vi "parse CSV files.vi"(6 "threshold cases":u32, 7 "SA data":T1, 8 "US data":T1, 9 "deaths CSV":string[][](array[string]), 10 "country index":u16, 11 "cases CSV":string[][](array[string])) -> (0 "new deaths per day":i32[](array[numeric]), 1 "days":i32[](array[numeric]), 2 "new cases per day":i32[](array[numeric]), 3 "first case date":timestamp, 4 "cumulative cases":i32[](array[numeric]), 5 "cumulative deaths":i32[](array[numeric]))   [LabVIEW 2019]
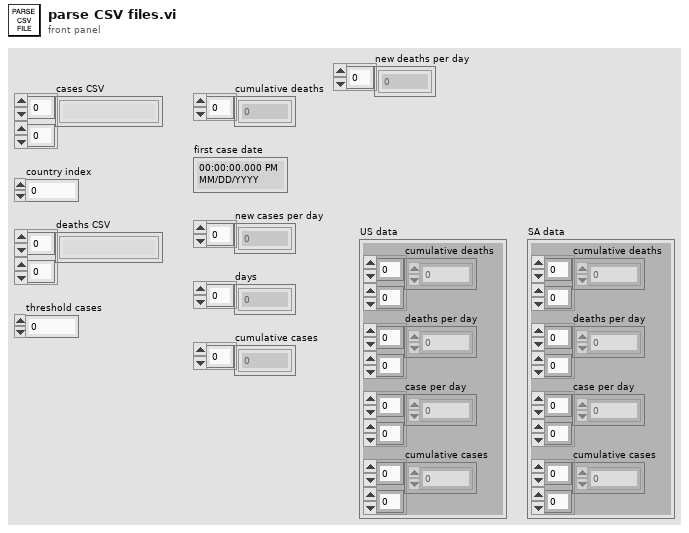
[diagram p1: front panel]
types:
  T1 = cluster{"cumulative deaths":i32[][], "deaths per day":i32[][], "case per day":i32[][], "cumulative cases":i32[][]}
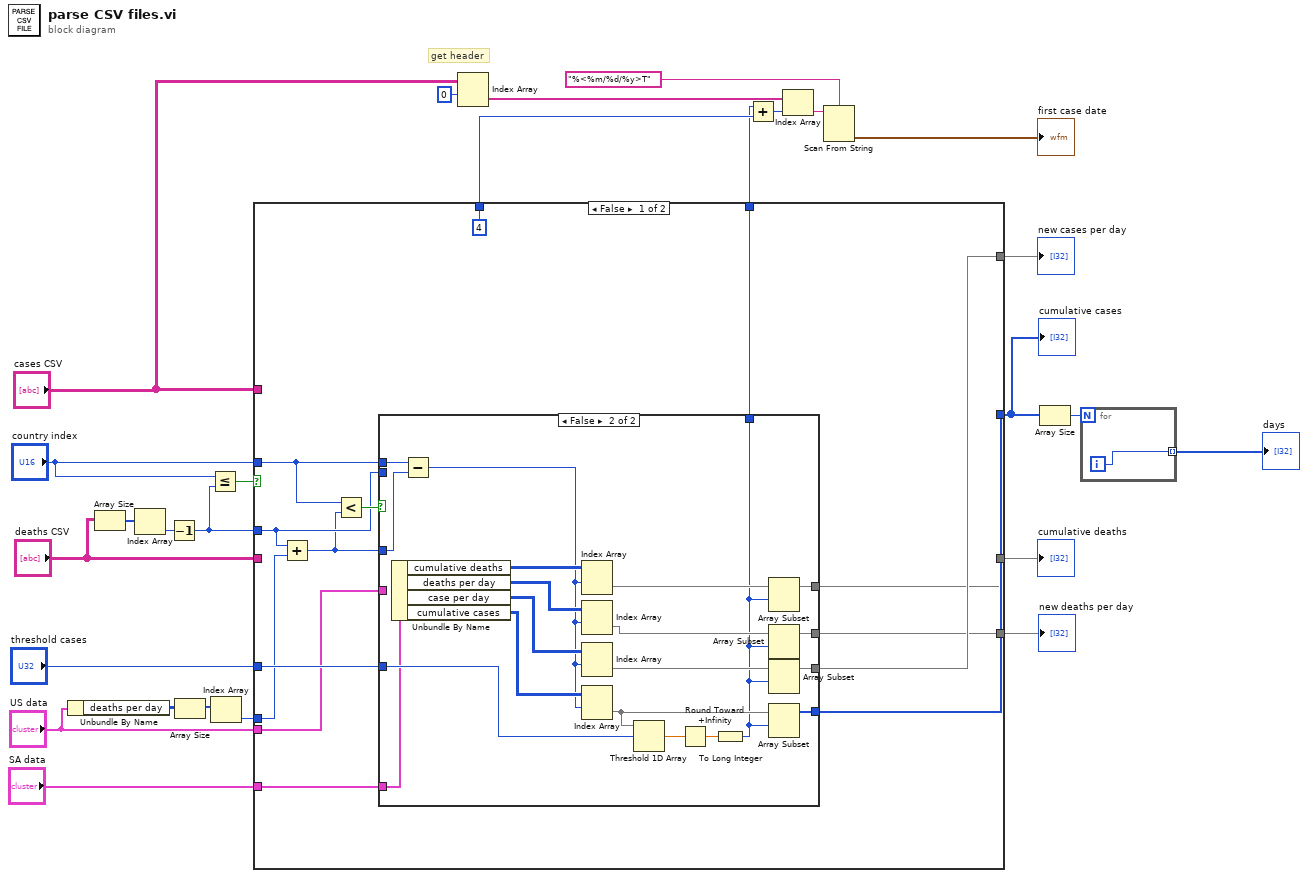
[diagram p0: block diagram]
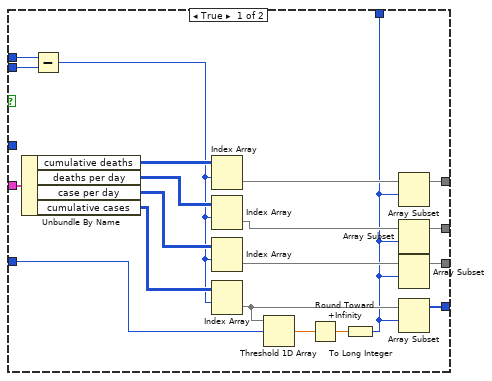
[diagram p2: hidden frame]
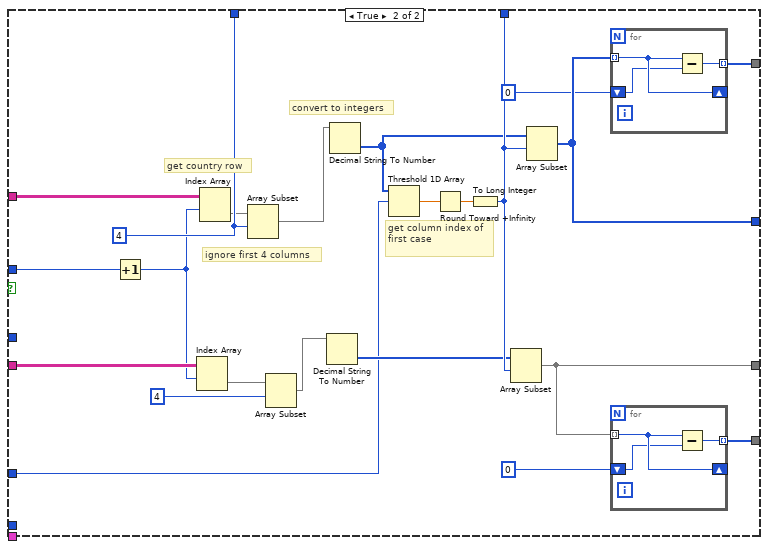
[diagram p3: hidden frame]
diagram:
  # "get header"
  n1 = Unbundle By Name("US data") -> ("deaths per day"=w3:i32[][])
  n2 = Array Size(array="deaths CSV") -> (size(s)=w9:i32[])
  n3 = Index Array(array=w9) -> (element=w8:i32)  [unwired: 1 in]
  n4 = Decrement(x=w8) -> (x-1=w7:i32)
  n5 = Array Size(array=w3) -> (size(s)=w2:i32[])
  n6 = Less Or Equal?(x="country index", y=w7) -> (x <= y?=w11:bool)
  n7 = Index Array(array=w2) -> (element=w1:i32)  [unwired: 1 in]
  n8 = case shown="False" w11 {
    tunnel: [4 ("index") w103] -> w26
    tunnel: [w35 w102] -> w25
    tunnel: "cases CSV" -> [_ w101]
    tunnel: "country index" -> [w28 w100]
    tunnel: "deaths CSV" -> [_ w99]
    tunnel: [w39 w95] -> w18
    tunnel: [w38 w94] -> w16
    tunnel: "threshold cases" -> [w40 w92]
    tunnel: [w36 w86] -> w13
    tunnel: [w37 w85] -> w12
    tunnel: "US data" -> [w31 _]
    tunnel: w7 -> [w33 _]
    tunnel: "SA data" -> [w30 _]
    tunnel: w1 -> [w32 _]
    frame False {
      n9 = Add(x=w33, y=w32) -> (x+y=w29:i32)
      n10 = Less?(x=w28, y=w29) -> (x < y?=w34:bool)
      n11 = case shown="False" w34 {
        tunnel: w31 -> [w61 _]
        tunnel: w40 -> [w50 w71]
        tunnel: [w49 w70] -> w39
        tunnel: [w48 w69] -> w38
        tunnel: [w47 w68] -> w37
        tunnel: [w46 w67] -> w36
        tunnel: [w45 w66] -> w35
        tunnel: w28 -> [w43 w64]
        tunnel: w33 -> [w42 _]
        tunnel: w30 -> [_ w63]
        tunnel: w29 -> [_ w62]
        frame True {
          n12 = Unbundle By Name(w61) -> ("cumulative deaths"=w60:i32[][], "deaths per day"=w59:i32[][], "case per day"=w58:i32[][], "cumulative cases"=w57:i32[][])
          n13 = Subtract(x=w43, y=w42) -> (x-y=w44:i32)
          n14 = Index Array(array=w60, index (row)=w44) -> (element=w56:i32[])  [unwired: 1 in]
          n15 = Index Array(array=w59, index (row)=w44) -> (element=w55:i32[])  [unwired: 1 in]
          n16 = Index Array(array=w58, index (row)=w44) -> (element=w54:i32[])  [unwired: 1 in]
          n17 = Index Array(array=w57, index (row)=w44) -> (element=w51:i32[])  [unwired: 1 in]
          n18 = Threshold 1D Array(2:w50, 3:w51) -> (0:w52:dbl)  [unwired: 1 in]
          n19 = Round Toward +Infinity(x=w52) -> (ceil(x): smallest int >= x=w53:dbl)
          n20 = To Long Integer(number=w53) -> (32bit integer=w45:i32)
          n21 = Array Subset(array=w56, index=w45) -> (w46:i32[])  [unwired: 1 in]
          n22 = Array Subset(array=w55, index=w45) -> (w47:i32[])  [unwired: 1 in]
          n23 = Array Subset(array=w54, index=w45) -> (w48:i32[])  [unwired: 1 in]
          n24 = Array Subset(array=w51, index=w45) -> (w49:i32[])  [unwired: 1 in]
        }
        frame False {
          n25 = Unbundle By Name(w63) -> ("cumulative deaths"=w81:i32[][], "deaths per day"=w80:i32[][], "case per day"=w79:i32[][], "cumulative cases"=w78:i32[][])
          n26 = Subtract(x=w64, y=w62) -> (x-y=w65:i32)
          n27 = Index Array(array=w81, index (row)=w65) -> (element=w77:i32[])  [unwired: 1 in]
          n28 = Index Array(array=w80, index (row)=w65) -> (element=w76:i32[])  [unwired: 1 in]
          n29 = Index Array(array=w79, index (row)=w65) -> (element=w75:i32[])  [unwired: 1 in]
          n30 = Index Array(array=w78, index (row)=w65) -> (element=w72:i32[])  [unwired: 1 in]
          n31 = Threshold 1D Array(2:w71, 3:w72) -> (0:w73:dbl)  [unwired: 1 in]
          n32 = Round Toward +Infinity(x=w73) -> (ceil(x): smallest int >= x=w74:dbl)
          n33 = To Long Integer(number=w74) -> (32bit integer=w66:i32)
          n34 = Array Subset(array=w77, index=w66) -> (w67:i32[])  [unwired: 1 in]
          n35 = Array Subset(array=w76, index=w66) -> (w68:i32[])  [unwired: 1 in]
          n36 = Array Subset(array=w75, index=w66) -> (w69:i32[])  [unwired: 1 in]
          n37 = Array Subset(array=w72, index=w66) -> (w70:i32[])  [unwired: 1 in]
        }
      }
    }
    frame True {
      w103 = 4 ("index")
      # "get column index of first case"
      # "convert to integers"
      # "ignore first 4 columns"
      # "get country row"
      n38 = Increment(x=w100) -> (x+1=w84:u16)
      n39 = Index Array(array=w99, index (row)=w84) -> (element=w96:string[])  [unwired: 1 in]
      n40 = Index Array(array=w101, index (row)=w84) -> (element=w88:string[])  [unwired: 1 in]
      n41 = Array Subset(array=w88, index=w103) -> (w82:string[])  [unwired: 1 in]
      n42 = Array Subset(array=w96, index=4) -> (w83:string[])  [unwired: 1 in]
      n43 = Decimal String To Number(string=w83) -> (number=w97:i32[])  [unwired: 2 in, 1 out]
      n44 = Decimal String To Number(string=w82) -> (number=w91:i32[])  [unwired: 2 in, 1 out]
      n45 = Threshold 1D Array(2:w92, 3:w91) -> (0:w89:dbl)  [unwired: 1 in]
      n46 = Round Toward +Infinity(x=w89) -> (ceil(x): smallest int >= x=w90:dbl)
      n47 = To Long Integer(number=w90) -> (32bit integer=w102:i32)
      n48 = Array Subset(array=w97, index=w102) -> (w86:i32[])  [unwired: 1 in]
      n49 = Array Subset(array=w91, index=w102) -> (w95:i32[])  [unwired: 1 in]
      n50 = for {
        tunnel: w95 -> [w109] mode=indexing
        shift-right: [w109] -> _
        shift-left: 0 -> [w108]
        tunnel: [w107] -> w94 mode=indexing
        n51 = Subtract(x=w109, y=w108) -> (x-y=w107:i32)
      }
      n52 = for {
        tunnel: w86 -> [w106] mode=indexing
        shift-right: [w106] -> _
        shift-left: 0 -> [w105]
        tunnel: [w104] -> w85 mode=indexing
        n53 = Subtract(x=w106, y=w105) -> (x-y=w104:i32)
      }
    }
  }
  "cumulative deaths" <- w13
  "cumulative cases" <- w18
  "new cases per day" <- w16
  "new deaths per day" <- w12
  n54 = Index Array(array="cases CSV", index (row)=0) -> (element=w23:string[])  [unwired: 1 in]
  n55 = Add(x=w25, y=w26) -> (x+y=w20:i32)
  n56 = Index Array(array=w23, index=w20) -> (element=w19:string)
  n57 = Scan From String(format string="%<%m/%d/%y>T", input string=w19) -> (output 1=→"first case date":timestamp)  [unwired: 3 in, 3 out]
  n58 = Array Size(array=w18) -> (size(s)=w14:i32)
  n59 = for {
    N: w14 -> [_]
    tunnel: [w110] -> w17 mode=indexing
    i -> [w110]
  }
  "days" <- w17
